vi "TestExec.Run Executable and Parse Results.vi"(6 "Reset":bool, 7 "Vars":variant, 8 "error in":errorcluster, 9 "Timeout(s)":dbl=500.0 caption="Time Out(s)" format="%.2f", 10 "Output Folder":path, 11 "Utility Config File":path) -> (0 "Error":errorcluster, 3 "RTN Data":T1 {"MeasData"."Status" items=["LOG", "PASS", "FAIL", "ERROR"]; "Attr"."Status" items=["LOG", "PASS", "FAIL", "ERROR"]; "Num"."Status" items=["LOG", "PASS", "FAIL", "ERROR"]})   [LabVIEW 2024]
uses:
  TestExec.Local Result Data.ctl
  Results/Result.Attribute.ctl
  Results/Result.Measurement and Attribute Item Status.ctl
  Results/Result.Numeric.ctl
  Results/Result.Limit Type.ctl
  Results/Result XML/TestResult.SW Item.ctl
  Reports/Report.Result FileDataObject.ctl
  Results/Result.Measurement Item.ctl
  Cmd Exe/CmdExe.Setup Params.ctl
  Cmd Exe/CmdExe.Output Error Check Setup.ctl
  <vilib>/Utility/error.llb/Trim Whitespace One-Sided.vi
  Errors.lvlib
  <vilib>/KATE/Time/Time Utils.lvlib
  <vilib>/KATE/Files/File Utils.lvlib
panel:
  in  "Tab Control":enum32{"Execute", "Results"}(tab)
  out "Active":bool
  out "Sys Exec Commands":string
  out "Sys Exec STDOut":string
  out "Dur(s)":dbl caption="Duration(s)" format="%.3f"
  out "Rslt":u32(colorbox)=13816530 caption="Exe"
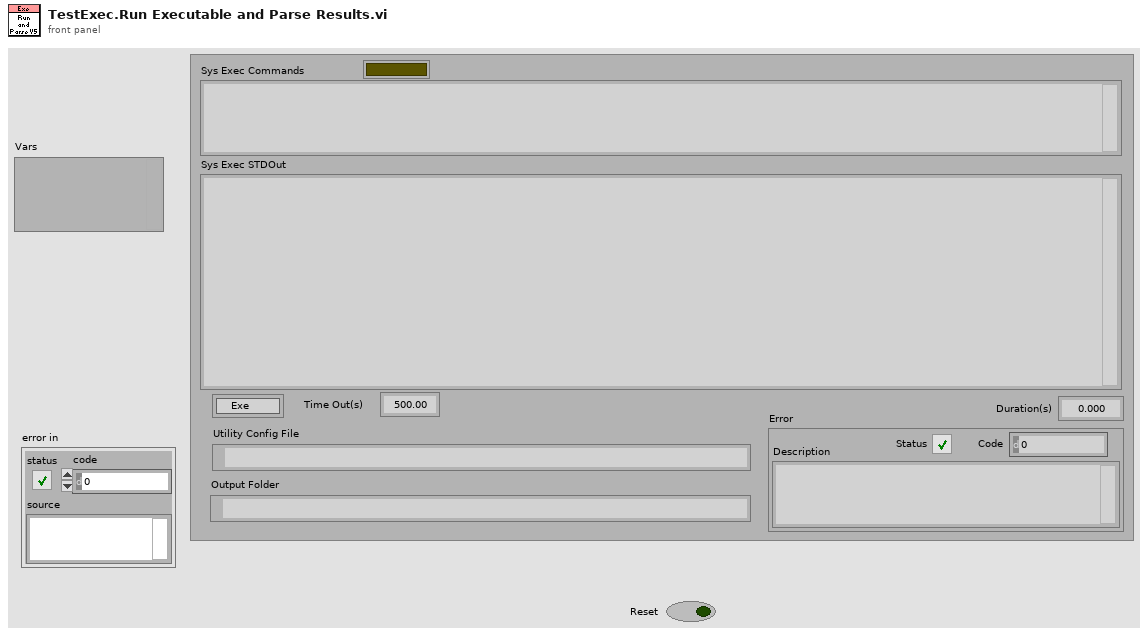
[diagram p1: front panel]
types:
  T1 = typedef "TestExec.Local Result Data.ctl" = cluster{"Attr":T2[], "Num":T4[], "UUT Props":string[][], "Vars":string[][], "SW Items":T6[], "Error":errorcluster, "Step":i32, "FileObjs":T7[], "MeasData":T8[]}
  T2 = typedef "Result.Attribute.ctl" = cluster{"Cnt":i32, "Step":string, "Category":string, "Name":string, "Value":string, "Status":T3, "Code":i32, "Desc":string, "Time":timestamp}
  T3 = typedef "Result.Measurement and Attribute Item Status.ctl" = i32
  T4 = typedef "Result.Numeric.ctl" = cluster{"Cnt":i32, "Step":string, "Category":string, "Name":string, "Value":dbl, "Units":string, "LimType":T5, "LL":dbl, "UL":dbl, "Status":T3, "Code":i32, "Desc":string, "Time":timestamp}
  T5 = typedef "Result.Limit Type.ctl" = enum16{"None", "EQ", "NE", "GT", "LT", "GE", "LE", "GTLT", "GELE", "GELT", "GTLE", "LTGT", "LEGE", "LEGT", "LTGE", "Contains", "NotContains"}
  T6 = typedef "TestResult.SW Item.ctl" = cluster{"Name":string, "PN":string, "Version":string, "Note":string}
  T7 = typedef "Report.Result FileDataObject.ctl" = cluster{"Cnt":i32, "Step":string, "Category":string, "Name":string, "Type":string, "File Name":string, "Time":string, "Path":path}
  T8 = typedef "Result.Measurement Item.ctl" = cluster{"Cnt":i32, "Step":string, "Category":string, "Name":string, "Value":string, "Units":string, "LimType":string, "LL":string, "UL":string, "Status":T3, "Code":i32, "Desc":string, "Time":timestamp}
  T9 = typedef "CmdExe.Setup Params.ctl" = cluster{"Timeout (s)":dbl, "Show Cmd Win":bool, "Error Check":T10, "Log_En":bool, "LogFileName":string, "LogDir":path}
  T10 = typedef "CmdExe.Output Error Check Setup.ctl" = cluster{"StdOut_Ck":bool, "StdOutErrMsgs":string[], "StdErr_Ck":bool, "RtnCode_Ck":bool, "RtnCodePASS":i32}
  T11 = cluster{"StdError":string, "RtnCode":i32, "Args":string, "Setup":T9, "StdOut":string, "ActionName":string, "Exe":path, "RTN Data":T1, "Prefix":string, "Code":i32, "OutputType":i32}
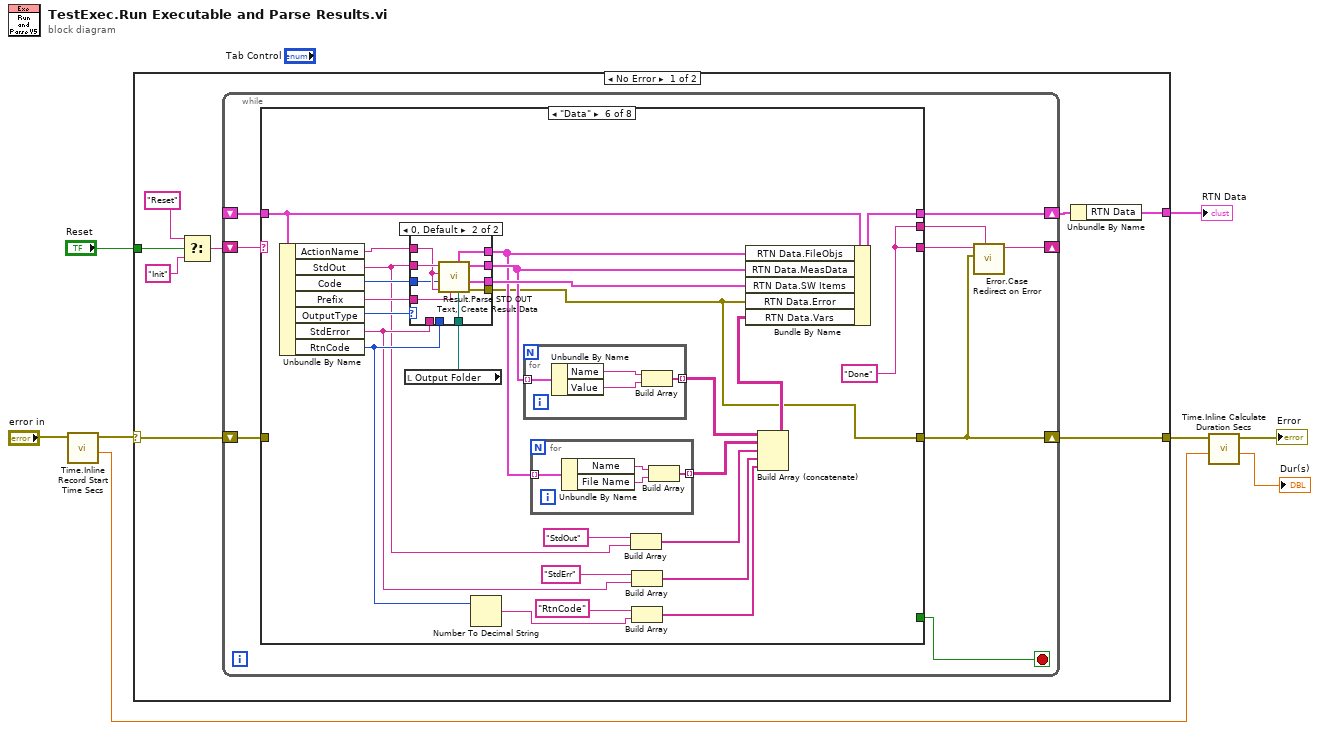
[diagram p0: block diagram]
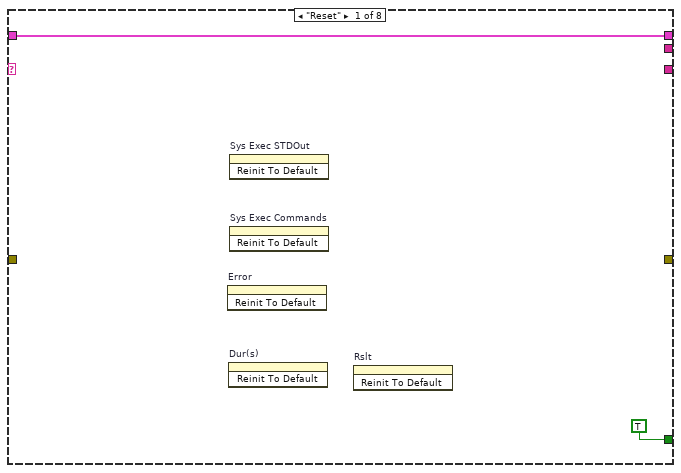
[diagram p2: hidden frame]
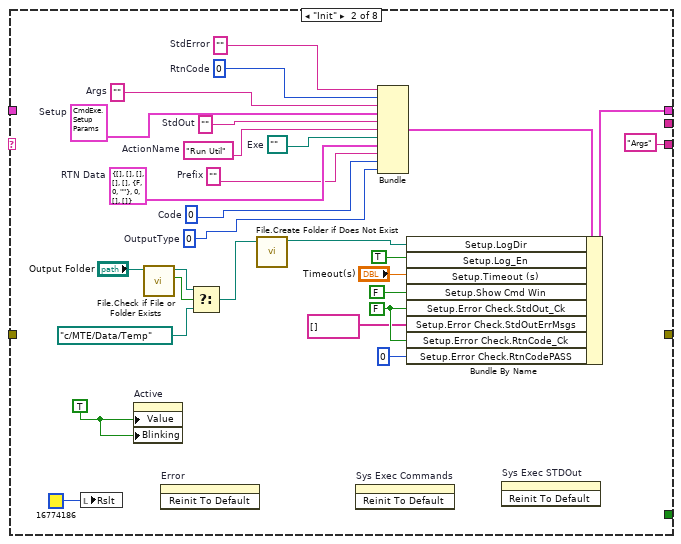
[diagram p3: hidden frame]
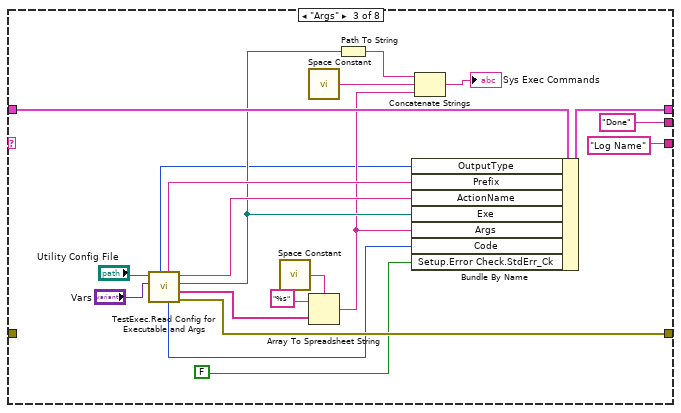
[diagram p4: hidden frame]
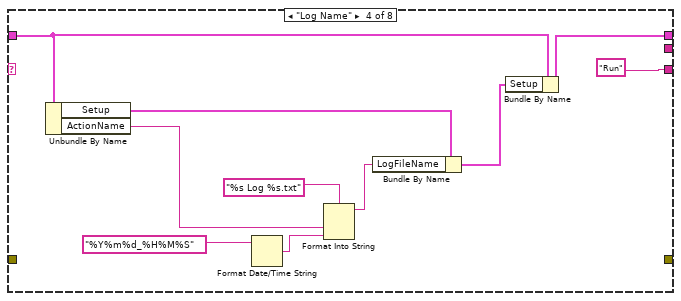
[diagram p5: hidden frame]
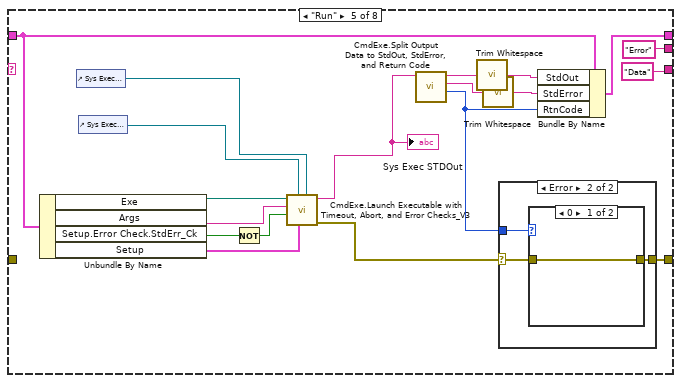
[diagram p6: hidden frame]
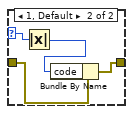
[diagram p8: hidden frame]
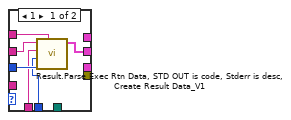
[diagram p9: hidden frame]
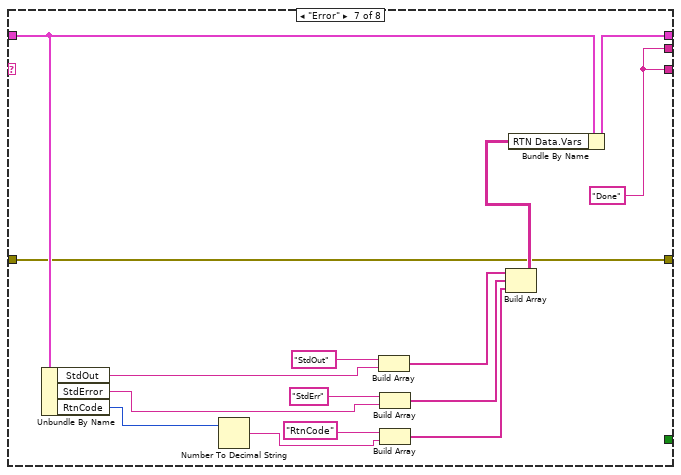
[diagram p10: hidden frame]
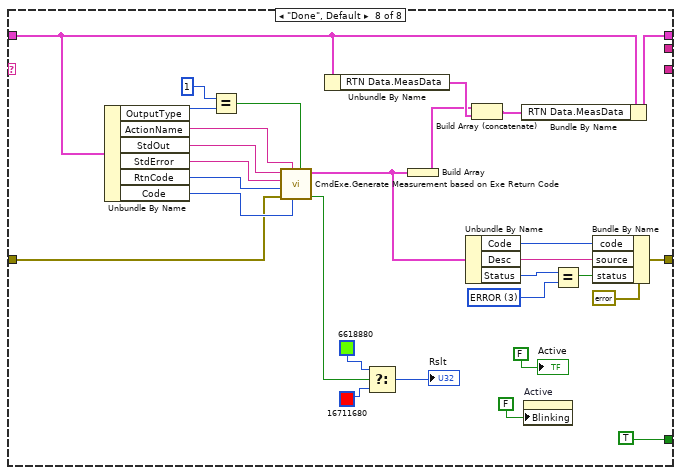
[diagram p11: hidden frame]
diagram:
  n1 = call <vilib>:"Time.Inline Record Start Time Secs.vi"("Error In Upper"="error in") -> ("Start(s)"=w2:dbl, "Error Out Upper"=w6:errorcluster)  [unwired: 8 in, 1 out]
  n2 = case shown="No Error" w6 {
    selector: w6 -> [w16 w205]
    tunnel: [w15 w205] -> w4
    tunnel: [w13 _] -> w8
    tunnel: "Reset" -> [w9 _]
    frame No Error {
      n3 = Select(t="Reset", s=w9, f="Init") -> (s? t:f=w11:string)
      n4 = while {
        shift-right: [w19] -> _
        shift-left: w11 -> [w25]
        shift-right: [w24] -> w14
        shift-left: _ -> [w23]
        shift-right: [w18] -> w15
        shift-left: w16 -> [w21]
        stop <- w22 stop-if-true
        n5 = case shown="\"Data\"" w25 {
          tunnel: [_ "Args" "Log Name" "Run" "Data" w113 w162 _] -> w20
          tunnel: [w27 w47 w75 w84 w96 w135 w175 w195] -> w24
          tunnel: w23 -> [w27 _ w74 w83 w91 w134 w174 w189]
          tunnel: [TRUE _ _ _ _ _ _ TRUE] -> w22
          tunnel: w21 -> [_ _ _ _ _ _ w161 w188]
          tunnel: [_ _ w67 _ w88 w127 w161 w180] -> w18
          tunnel: [_ _ "Done" ("Error Case") _ "Error" w113 w162 _] -> w17
          frame "Reset" {
            n6 = invoke on="Error" class="Clust (strict)" method="Reinit To Default"() -> ()  [unwired: 3 in, 3 out]
            n7 = invoke on="Dur(s)" class="DigNum (strict)" method="Reinit To Default"() -> ()  [unwired: 3 in, 3 out]
            n8 = invoke on="Sys Exec STDOut" class="Str" method="Reinit To Default"() -> ()  [unwired: 3 in, 3 out]
            n9 = invoke on="Sys Exec Commands" class="Str" method="Reinit To Default"() -> ()  [unwired: 3 in, 3 out]
            n10 = invoke on="Rslt" class="ColBox" method="Reinit To Default"() -> ()  [unwired: 3 in, 3 out]
          }
          frame "Init" {
            w36 = 0  # RtnCode
            w35 = ""  # StdError
            w37 = 0  # OutputType
            w38 = 0  # Code
            w39 = ""  # Prefix
            w40 = T1 {"Attr"=[], "Num"=[], "UUT Props"=[], "Vars"=[], "SW Items"=[], "Error"={"status"=FALSE, "code"=0, "source"=""}, "Step"=0, "FileObjs"=[], "MeasData"=[]}  # RTN Data
            w41 = path ""  # Exe
            w42 = "Run Util"  # ActionName
            w44 = ""  # StdOut
            w48 = FALSE
            w53 = TRUE ("Value")
            w52 = T9 {"Timeout (s)"=60.0, "Show Cmd Win"=FALSE, "Error Check"={"StdOut_Ck"=FALSE, "StdOutErrMsgs"=["Error", "Unable to find device "], "StdErr_Ck"=FALSE, "RtnCode_Ck"=FALSE, "RtnCodePASS"=0}, "Log_En"=FALSE, "LogFileName"="", "LogDir"=path ""}  # Setup
            w55 = ""  # Args
            n11 = local write "Rslt"(u32 16774186) -> ()
            n12 = property on="Active" class="Bool (strict)"("Value"=w53, "Blinking"=w53) -> ()  [unwired: 2 in, 2 out]
            n13 = call <vilib>:"File.Check if File or Folder Exists.vi"("Path"="Output Folder") -> ("Exists"=w31:bool, "Dup Path"=w32:path)  [unwired: 6 in, 3 out]
            n14 = invoke on="Error" class="Clust (strict)" method="Reinit To Default"() -> ()  [unwired: 3 in, 3 out]
            n15 = Select(t=w32, s=w31, f=path "c:/MTE/Data/Temp") -> (s? t:f=w29:path)
            n16 = call <vilib>:"File.Create Folder if Does Not Exist.vi"("Path"=w29) -> ("Dup Path"=w28:path)  [unwired: 8 in, 2 out]
            n17 = invoke on="Sys Exec Commands" class="Str" method="Reinit To Default"() -> ()  [unwired: 3 in, 3 out]
            n18 = Bundle("StdError"=w35, "RtnCode"=w36, "Args"=w55, "Setup"=w52, "StdOut"=w44, "ActionName"=w42, "Exe"=w41, "RTN Data"=w40, "Prefix"=w39, "Code"=w38, "OutputType"=w37) -> (w49:T11)  [unwired: 1 in]
            n19 = Bundle By Name(cluster=w49, "Setup.LogDir"=w28, "Setup.Log_En"=TRUE, "Setup.Timeout (s)"="Timeout(s)", "Setup.Show Cmd Win"=FALSE, "Setup.Error Check.StdOut_Ck"=w48, "Setup.Error Check.StdOutErrMsgs"=string[] [], "Setup.Error Check.RtnCode_Ck"=w48, "Setup.Error Check.RtnCodePASS"=0 ("Error Check.RtnCodePASS")) -> (w47:T11)
            n20 = invoke on="Sys Exec STDOut" class="Str" method="Reinit To Default"() -> ()  [unwired: 3 in, 3 out]
          }
          frame "Args" {
            n21 = call "TestExec.Read Config for Executable and Args.vi"("Vars"="Vars", "Config File"="Utility Config File") -> ("error out"=w67:errorcluster, "Args"=w69:string[], "Exe"=w61:path, "Action Name"=w66:string, "Error Code"=w65:i32, "Data Name Prefix"=w64:string, "OutType"=w57:i32)  [unwired: 2 in, 1 out]
            n22 = call <vilib>:"Space Constant.vi"() -> ("String"=w70:string)
            n23 = call <vilib>:"Space Constant.vi"() -> ("String"=w59:string)
            n24 = Array To Spreadsheet String(delimiter (Tab)=w70, array=w69, 3:"%s" ("format string")) -> (spreadsheet string=w60:string)
            n25 = Path To String(path=w61) -> (string=w62:string)
            n26 = Bundle By Name(cluster=w74, "OutputType"=w57, "Prefix"=w64, "ActionName"=w66, "Exe"=w61, "Args"=w60, "Code"=w65, "Setup.Error Check.StdErr_Ck"=FALSE) -> (w75:T11)
            n27 = Concatenate Strings(w62, w59, w60) -> (→"Sys Exec Commands":string)
          }
          frame "Log Name" {
            n28 = Unbundle By Name(w83) -> ("Setup"=w81:T9, "ActionName"=w76:string)
            n29 = Format Date/Time String(time format string (%c)="%Y%m%d_%H%M%S") -> (date/time string=w77:string)  [unwired: 2 in]
            n30 = Format Into String(format string="%s Log %s.txt", w76, w77) -> (resulting string=w78:string)  [unwired: 2 in, 1 out]
            n31 = Bundle By Name(cluster=w81, "LogFileName"=w78) -> (w82:T9)
            n32 = Bundle By Name(cluster=w83, "Setup"=w82) -> (w84:T11)
          }
          frame "Run" {
            n33 = Unbundle By Name(w91) -> ("Exe"=w97:path, "Args"=w104:string, "Setup.Error Check.StdErr_Ck"=w95:bool, "Setup"=w103:T9)
            n34 = control-ref of="Sys Exec Commands"() -> (w102:refnum<vi>)
            n35 = control-ref of="Sys Exec STDOut"() -> (w101:refnum<vi>)
            n36 = Not(x=w95) -> (.not. x?=w94:bool)
            n37 = call "CmdExe.Launch Executable with Timeout, Abort, and Error Checks_V3.vi"("Cmd IN Ref"=w102, "Setup"=w103, "Output Ref"=w101, "Ignore StdErr"=w94, "Args"=w104, "Executable"=w97) -> ("error out"=w90:errorcluster, "Data Out"=w99:string)  [unwired: 2 in, 2 out]
            "Sys Exec STDOut" <- w99
            n38 = call "CmdExe.Split Output Data to StdOut, StdError, and Return Code.vi"("Output Data"=w99) -> ("Return Code"=w89:i32, "StdError"=w93:string, "StdOut"=w100:string)  [unwired: 7 in, 1 out]
            n39 = call <vilib>:"Trim Whitespace.vi"("string"=w100) -> ("trimmed string"=w98:string)  [unwired: 1 in]
            n40 = call <vilib>:"Trim Whitespace.vi"("string"=w93) -> ("trimmed string"=w92:string)  [unwired: 1 in]
            n41 = case shown="Error" w90 {
              selector: w90 -> [_ w106]
              tunnel: w89 -> [_ w107]
              tunnel: [_ w105] -> w88
              frame No Error {
              }
              frame Error {
                n42 = case shown="0" w107 {
                  selector: w107 -> [_ w112]
                  tunnel: w106 -> [w108 w111]
                  tunnel: [w108 w110] -> w105
                  frame 0 {
                  }
                  frame 1, Default {
                    n43 = Absolute Value(x=w112) -> (abs(x)=w109:i32)
                    n44 = Bundle By Name(cluster=w111, "code"=w109) -> (w110:errorcluster)
                  }
                }
              }
            }
            n45 = Bundle By Name(cluster=w91, "StdOut"=w98, "StdError"=w92, "RtnCode"=w89) -> (w96:T11)
          }
          frame "Data" {
            w113 = "Done"
            n46 = Unbundle By Name(w134) -> ("ActionName"=w131:string, "StdOut"=w114:string, "Code"=w126:i32, "Prefix"=w125:string, "OutputType"=w124:i32, "StdError"=w115:string, "RtnCode"=w117:i32)
            n47 = local read "Output Folder"() -> (w136:path)
            n48 = case shown="0, Default" w124 {
              tunnel: w114 -> [w142 w152]
              tunnel: [_ w151] -> w137
              tunnel: w136 -> [_ w150]
              tunnel: [w140 w149] -> w133
              tunnel: [_ w148] -> w132
              tunnel: w131 -> [w141 w147]
              tunnel: [_ w146] -> w127
              tunnel: w126 -> [w143 w145]
              tunnel: w125 -> [_ w144]
              tunnel: w115 -> [w139 _]
              tunnel: w117 -> [w138 _]
              frame 1 {
                n49 = call "Result.Parse Exec Rtn Data, STD OUT is code, Stderr is desc, Create Result Data_V1.vi"("Name"=w141, "BaseCode"=w143, "RtnCode"=w138, "StdErr"=w139, "StdOut"=w142) -> ("Meas"=w140:T8[])  [unwired: 6 in]
              }
              frame 0, Default {
                n50 = call "Result.Parse STD OUT Text, Create Result Data.vi"("UUTDir"=w150, "Prefix"=w144, "Version Name"=w147, "Error Code"=w145, "Task Name"=w147, "StdOut"=w152) -> ("Error"=w146:errorcluster, "SW Ver"=w151:T6[], "Meas"=w149:T8[], "Data Files"=w148:T7[])  [unwired: 2 in]
              }
            }
            n51 = Number To Decimal String(number=w117) -> (decimal integer string=w116:string)  [unwired: 1 in]
            n52 = for {
              tunnel: w133 -> [w160] mode=indexing
              tunnel: [w157] -> w130 mode=indexing
              n53 = Unbundle By Name(w160) -> ("Name"=w159:string, "Value"=w158:string)
              n54 = Build Array(w159, w158) -> (w157:string[])
            }
            n55 = for {
              tunnel: w132 -> [w156] mode=indexing
              tunnel: [w154] -> w129 mode=indexing
              n56 = Unbundle By Name(w156) -> ("Name"=w155:string, "File Name"=w153:string)
              n57 = Build Array(w155, w153) -> (w154:string[])
            }
            n58 = Build Array("StdOut", w114) -> (w122:string[])
            n59 = Build Array("StdErr", w115) -> (w121:string[])
            n60 = Build Array("RtnCode", w116) -> (w118:string[])
            n61 = Build Array (concatenate)(w130, w129, w122, w121, w118) -> (w128:string[][])
            n62 = Bundle By Name(cluster=w134, "RTN Data.FileObjs"=w132, "RTN Data.MeasData"=w133, "RTN Data.SW Items"=w137, "RTN Data.Error"=w127, "RTN Data.Vars"=w128) -> (w135:T11)
          }
          frame "Error" {
            w162 = "Done"
            n63 = Unbundle By Name(w174) -> ("StdOut"=w163:string, "StdError"=w164:string, "RtnCode"=w166:i32)
            n64 = Number To Decimal String(number=w166) -> (decimal integer string=w165:string)  [unwired: 1 in]
            n65 = Build Array("StdOut", w163) -> (w171:string[])
            n66 = Build Array("StdErr", w164) -> (w170:string[])
            n67 = Build Array("RtnCode", w165) -> (w167:string[])
            n68 = Build Array(w171, w170, w167) -> (w173:string[][])
            n69 = Bundle By Name(cluster=w174, "RTN Data.Vars"=w173) -> (w175:T11)
          }
          frame "Done", Default {
            w182 = T3 3 items=["LOG", "PASS", "FAIL", "ERROR"] ("Status")
            n70 = Unbundle By Name(w189) -> ("OutputType"=w178:i32, "ActionName"=w194:string, "StdOut"=w193:string, "StdError"=w192:string, "RtnCode"=w191:i32, "Code"=w190:i32)
            n71 = Equal?(x=1, y=w178) -> (x = y?=w176:bool)
            n72 = call "CmdExe.Generate Measurement based on Exe Return Code.vi"("StdOut is Fail Code"=w176, "BaseCode"=w190, "Name"=w194, "Error"=w188, "RtnCode"=w191, "StdErr"=w192, "StdOut"=w193) -> ("Success"=w187:bool, "Meas"=w179:T8)  [unwired: 3 in]
            n73 = Unbundle By Name(w189) -> ("RTN Data.MeasData"=w198:T8[])
            n74 = Select(t=u32 6618880, s=w187, f=u32 16711680) -> (s? t:f=→"Rslt":u32)
            n75 = Build Array(w179) -> (w197:T8[])
            n76 = Unbundle By Name(w179) -> ("Code"=w184:i32, "Desc"=w185:string, "Status"=w183:T3)
            n77 = Build Array (concatenate)(w197, w198) -> (w199:T8[])
            n78 = Bundle By Name(cluster=w189, "RTN Data.MeasData"=w199) -> (w195:T11)
            n79 = property on="Active" class="Bool (strict)"("Blinking"=FALSE ("Value")) -> ()  [unwired: 2 in, 2 out]
            n80 = Equal?(x=w183, y=w182) -> (x = y?=w181:bool)
            n81 = Bundle By Name(cluster=errorcluster {"status"=FALSE, "code"=0, "source"=""} ("error constant"), "code"=w184, "source"=w185, "status"=w181) -> (w180:errorcluster)
            "Active" <- FALSE ("Active")
          }
        }
        n82 = call "Error.Case Redirect on Error.vi"("Error Case"=w17, "error in"=w18, "Next Case"=w20) -> ("Next Case Out"=w19:string)  [unwired: 8 in]
      }
      n83 = Unbundle By Name(w14) -> ("RTN Data"=w13:T1)
    }
    frame Error {
    }
  }
  "RTN Data" <- w8
  n84 = call <vilib>:"Time.Inline Calculate Duration Secs.vi"("Start(Sec)"=w2, "Error In Top"=w4) -> ("Duration(s)"=→"Dur(s)":dbl, "Error Out Top"=→"Error":errorcluster)  [unwired: 7 in, 1 out]
